vi "Read speed.vi"(11 "shooter in":refnum<class "shooter.lvclass">) -> (2 "speed":dbl, 3 "shooter out":refnum<class "shooter.lvclass">)   [LabVIEW 2015, in "shooter.lvclass"]
uses:
  shooter.lvclass
  shooter.lvclass/shooter.ctl
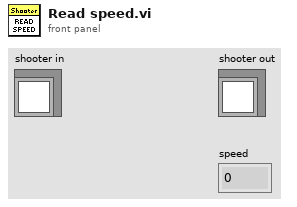
[diagram p1: front panel]
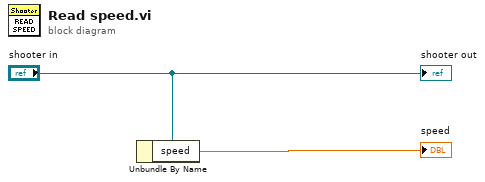
[diagram p0: block diagram]
diagram:
  n1 = Unbundle By Name("shooter in") -> ("speed"=→"speed":dbl)
  "shooter out" <- "shooter in"
